vi "read config.vi"(8 "error in (no error)":errorcluster, 10 "file path (use dialog)":path, 11 "general in":refnum<class "general.lvclass">) -> (0 "error out":errorcluster, 3 "general out":refnum<class "general.lvclass">)   [LabVIEW 2025, in "general.lvclass"]
uses:
  general.lvclass
  general.lvclass/general.ctl
  74c86caf-b241-4b61-b29c-35602bed4a9e.vi
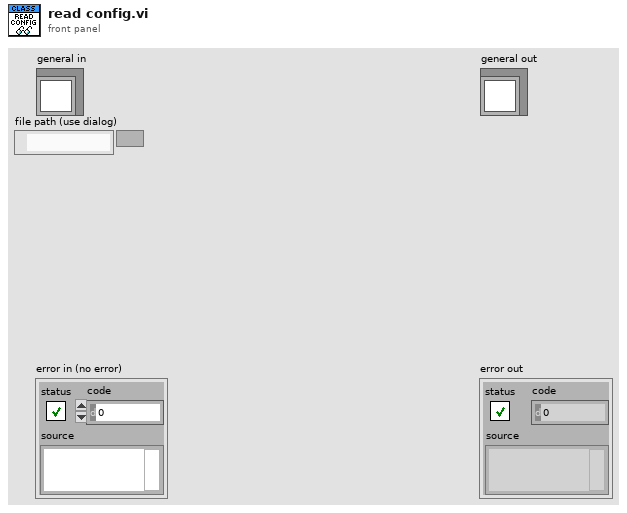
[diagram p1: front panel]
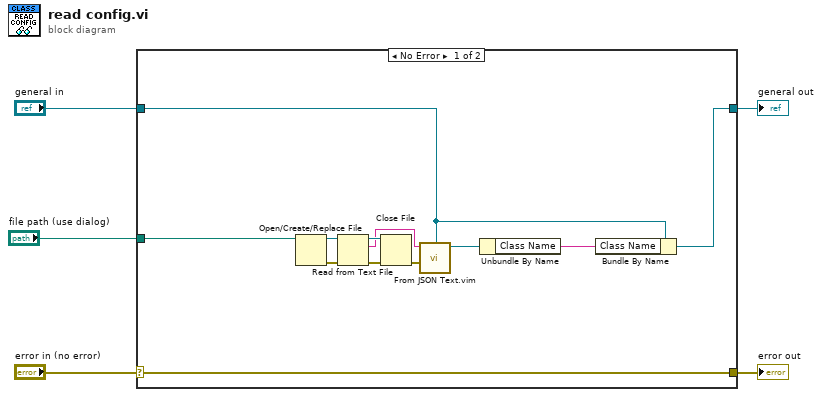
[diagram p0: block diagram]
diagram:
  n1 = case shown="No Error" "error in (no error)" {
    selector: "error in (no error)" -> [w17 w19]
    tunnel: [w17 w19] -> w4
    tunnel: [w6 w18] -> w2
    tunnel: "general in" -> [w7 w18]
    tunnel: "file path (use dialog)" -> [w10 _]
    frame No Error {
      n2 = Open/Create/Replace File(file path (use dialog)=w10) -> (refnum out=w13:refnum<file>, error out=w16:errorcluster)  [unwired: 5 in, 1 out]
      n3 = Read from Text File(file (use dialog)=w13, error in=w16) -> (refnum out=w14:refnum<file>, text=w12:string, error out=w15:errorcluster)  [unwired: 2 in, 1 out]
      n4 = Close File(refnum=w14, error in=w15) -> (error out=w11:errorcluster)  [unwired: 1 out]
      n5 = call "From JSON Text.vim"("Data Type and Default Value"=w7, "error in (no error)"=w11, "JSON"=w12) -> ("Data out"=w9:refnum<class "general.lvclass">)  [unwired: 7 in, 1 out]
      n6 = Unbundle By Name(w9) -> ("Class Name"=w8:string)
      n7 = Bundle By Name(cluster=w7, "Class Name"=w8) -> (w6:refnum<class "general.lvclass">)
    }
    frame Error {
    }
  }
  "error out" <- w4
  "general out" <- w2
